vi "1-1 이벤트핸들러.vi"() -> ()   [LabVIEW 2014]
uses:
  <vilib>/Analysis/1siggen.llb/General Aperiodic Triangle.vi
  <vilib>/Analysis/NI_AALBase.lvlib
panel:
  out "시간":u32
  out "웨이브폼 그래프":dbl[](graph)
  in  "삼각":bool
  in  "정지":bool
  in  "Sine":bool
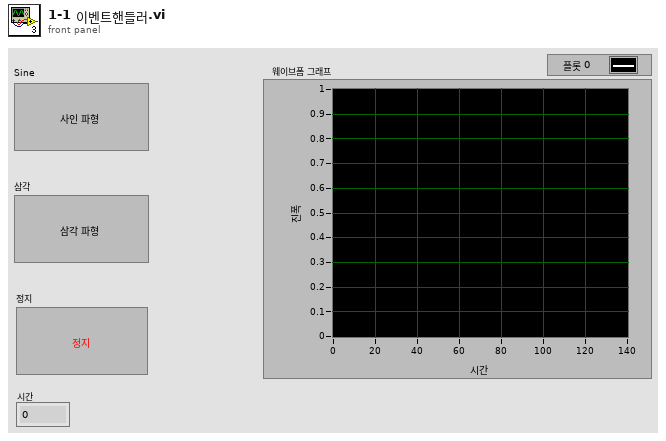
[diagram p1: front panel]
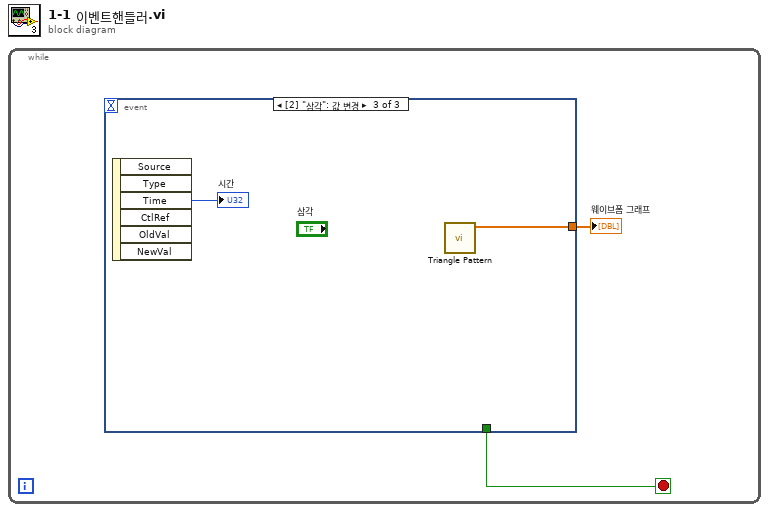
[diagram p0: block diagram]
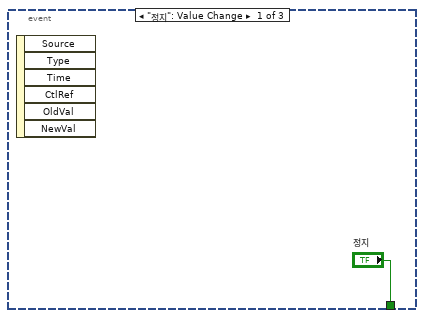
[diagram p2: hidden frame]
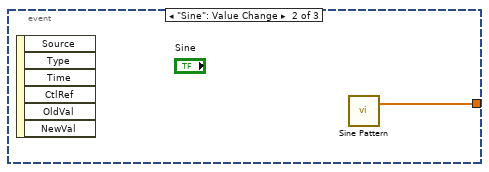
[diagram p3: hidden frame]
diagram:
  n1 = while {
    stop <- w2 stop-if-true
    n2 = event shown="[2] \"삼각\": 값 변경" {
      selector: _ -> [_ _ _]
      dyn-events: _ -> [_ _ _]
      timeout: _ -> [_ _ _]
      tunnel: ["정지" _ _] -> w2
      tunnel: [_ w4 w6] -> w1
      event "정지": Value Change {
        n3 = event-data() -> ()  [unwired: 1 in, 6 out]
      }
      event "Sine": Value Change {
        n4 = event-data() -> ()  [unwired: 1 in, 6 out]
        n5 = call <vilib>:"Sine Pattern.vi"() -> ("Sinusoidal Pattern"=w4:dbl[])  [unwired: 4 in, 1 out]
      }
      event "삼각": Value Change {
        n6 = event-data() -> ("Time"=→"시간":u32)  [unwired: 1 in, 5 out]
        n7 = call <vilib>:"Triangle Pattern.vi"() -> ("Triangle Pattern"=w6:dbl[])  [unwired: 10 in, 1 out]
      }
    }
    "웨이브폼 그래프" <- w1
  }
